vi "PID Drive.vi"(6 "Rotation":dbl, 7 "Gyro Angle":dbl, 8 "error in (no error)":errorcluster, 9 "Y":dbl, 10 "X":dbl, 11 "RobotDriveDevRef 2":T2={"DevStatus"={"status"=FALSE, "code"=0, "source"=""}, "Motors[]"=[{"DeviceStatus"={"status"=FALSE, "code"=0, "source"=""}, "Type"=enum."PWM", "PWM"={"Digital Module"=enum."Digital Module 1", "PWM Channel"=enum."PWM 2", "DeadBand"={"Name"="Victor", "maxPositivePwm"=208, "minPositivePwm"=129, "centerPwm"=128, "maxNegativePwm"=127, "minNegativePwm"=54, "angularRange"=0}}, "CAN"={"Device Number"=0, "Control Mode"=enum."Percent VBus", "Semaphore"=refnum, "Max Vout"=0.0}, "Invert"=FALSE, "TransformRef"=refnum, "InvTransformRef"=refnum}, {"DeviceStatus"={"status"=FALSE, "code"=0, "source"=""}, "Type"=enum."PWM", "PWM"={"Digital Module"=enum."Digital Module 1", "PWM Channel"=enum."PWM 1", "DeadBand"={"Name"="Victor", "maxPositivePwm"=208, "minPositivePwm"=129, "centerPwm"=128, "maxNegativePwm"=127, "minNegativePwm"=54, "angularRange"=0}}, "CAN"={"Device Number"=0, "Control Mode"=enum."Percent VBus", "Semaphore"=refnum, "Max Vout"=0.0}, "Invert"=TRUE, "TransformRef"=refnum, "InvTransformRef"=refnum}, {"DeviceStatus"={"status"=FALSE, "code"=0, "source"=""}, "Type"=enum."PWM", "PWM"={"Digital Module"=enum."Digital Module 1", "PWM Channel"=enum."PWM 4", "DeadBand"={"Name"="Victor", "maxPositivePwm"=208, "minPositivePwm"=129, "centerPwm"=128, "maxNegativePwm"=127, "minNegativePwm"=54, "angularRange"=0}}, "CAN"={"Device Number"=0, "Control Mode"=enum."Percent VBus", "Semaphore"=refnum, "Max Vout"=0.0}, "Invert"=FALSE, "TransformRef"=refnum, "InvTransformRef"=refnum}, {"DeviceStatus"={"status"=FALSE, "code"=0, "source"=""}, "Type"=enum."PWM", "PWM"={"Digital Module"=enum."Digital Module 1", "PWM Channel"=enum."PWM 3", "DeadBand"={"Name"="Victor", "maxPositivePwm"=208, "minPositivePwm"=129, "centerPwm"=128, "maxNegativePwm"=127, "minNegativePwm"=54, "angularRange"=0}}, "CAN"={"Device Number"=0, "Control Mode"=enum."Percent VBus", "Semaphore"=refnum, "Max Vout"=0.0}, "Invert"=TRUE, "TransformRef"=refnum, "InvTransformRef"=refnum}], "Square Inputs"=TRUE, "Max Output"=1.0, "Isochronous"=FALSE}) -> (0 "error out":errorcluster, 2 "Motor Values":dbl[](array[numeric])=[0.0, -0.0, 0.0, -0.0], 3 "RobotDriveDevRef":T2={"DevStatus"={"status"=FALSE, "code"=0, "source"=""}, "Motors[]"=[{"DeviceStatus"={"status"=FALSE, "code"=0, "source"=""}, "Type"=enum."PWM", "PWM"={"Digital Module"=enum."Digital Module 1", "PWM Channel"=enum."PWM 2", "DeadBand"={"Name"="Victor", "maxPositivePwm"=208, "minPositivePwm"=129, "centerPwm"=128, "maxNegativePwm"=127, "minNegativePwm"=54, "angularRange"=0}}, "CAN"={"Device Number"=0, "Control Mode"=enum."Percent VBus", "Semaphore"=refnum, "Max Vout"=0.0}, "Invert"=FALSE, "TransformRef"=refnum, "InvTransformRef"=refnum}, {"DeviceStatus"={"status"=FALSE, "code"=0, "source"=""}, "Type"=enum."PWM", "PWM"={"Digital Module"=enum."Digital Module 1", "PWM Channel"=enum."PWM 1", "DeadBand"={"Name"="Victor", "maxPositivePwm"=208, "minPositivePwm"=129, "centerPwm"=128, "maxNegativePwm"=127, "minNegativePwm"=54, "angularRange"=0}}, "CAN"={"Device Number"=0, "Control Mode"=enum."Percent VBus", "Semaphore"=refnum, "Max Vout"=0.0}, "Invert"=TRUE, "TransformRef"=refnum, "InvTransformRef"=refnum}, {"DeviceStatus"={"status"=FALSE, "code"=0, "source"=""}, "Type"=enum."PWM", "PWM"={"Digital Module"=enum."Digital Module 1", "PWM Channel"=enum."PWM 4", "DeadBand"={"Name"="Victor", "maxPositivePwm"=208, "minPositivePwm"=129, "centerPwm"=128, "maxNegativePwm"=127, "minNegativePwm"=54, "angularRange"=0}}, "CAN"={"Device Number"=0, "Control Mode"=enum."Percent VBus", "Semaphore"=refnum, "Max Vout"=0.0}, "Invert"=FALSE, "TransformRef"=refnum, "InvTransformRef"=refnum}, {"DeviceStatus"={"status"=FALSE, "code"=0, "source"=""}, "Type"=enum."PWM", "PWM"={"Digital Module"=enum."Digital Module 1", "PWM Channel"=enum."PWM 3", "DeadBand"={"Name"="Victor", "maxPositivePwm"=208, "minPositivePwm"=129, "centerPwm"=128, "maxNegativePwm"=127, "minNegativePwm"=54, "angularRange"=0}}, "CAN"={"Device Number"=0, "Control Mode"=enum."Percent VBus", "Semaphore"=refnum, "Max Vout"=0.0}, "Invert"=TRUE, "TransformRef"=refnum, "InvTransformRef"=refnum}], "Square Inputs"=TRUE, "Max Output"=1.0, "Isochronous"=FALSE})   [LabVIEW 2013]
uses:
  <vilib>/Rock Robotics/WPI/RobotDrive/WPI_RobotDriveDevRef.ctl
  <vilib>/Rock Robotics/WPI/MotorControl/WPI_MotorControlDeviceRef.ctl
  <vilib>/Rock Robotics/SystemInterfaces/Typedef/FPGA_TypedefDigitalModule.ctl
  <vilib>/Rock Robotics/SystemInterfaces/DIO/FPGA_DIOPWMChannel.ctl
  <vilib>/Rock Robotics/WPI/PWM/WPI_PWMDeadband.ctl
  <vilib>/Rock Robotics/WPI/CAN/Jaguar/SubVIs/WPI_CANJaguar_ControlMode.ctl
  <vilib>/Rock Robotics/WPI/PWM/WPI_PWMTransform_ConPane.ctl
  <vilib>/Rock Robotics/SystemInterfaces/NetworkCommunication/NetComm_UsageReport_ResourceType.ctl
  <vilib>/Rock Robotics/WPI/RobotDrive/WPI_RobotDriveMotorSelectorEnum.ctl
  <vilib>/addons/control/pid/pid.llb/PID (DBL).vi
  <vilib>/Rock Robotics/WPI/RobotDrive/WPI_RobotDriveSafetyCheck.vi
  <vilib>/addons/control/pid/NI_PID_pid.lvlib
panel:
  in  "Encoder Max":dbl=200.0
  in  "Back Right":T1={"proportional gain (Kc)"=0.01, "integral time (Ti, min)"=0.0, "derivative time (Td, min)"=0.0} {"derivative time (Td, min)" format="%.3f"; "integral time (Ti, min)" format="%.3f"; "proportional gain (Kc)" format="%.3f"}
  in  "Front Right":T1={"proportional gain (Kc)"=1.0, "integral time (Ti, min)"=0.0, "derivative time (Td, min)"=0.0} {"derivative time (Td, min)" format="%.3f"; "integral time (Ti, min)" format="%.3f"; "proportional gain (Kc)" format="%.3f"}
  in  "Back Left":T1={"proportional gain (Kc)"=0.01, "integral time (Ti, min)"=0.0, "derivative time (Td, min)"=0.0} {"derivative time (Td, min)" format="%.3f"; "integral time (Ti, min)" format="%.3f"; "proportional gain (Kc)" format="%.3f"}
  in  "Front Left":T1={"proportional gain (Kc)"=0.01, "integral time (Ti, min)"=0.0, "derivative time (Td, min)"=0.0} {"derivative time (Td, min)" format="%.3f"; "integral time (Ti, min)" format="%.3f"; "proportional gain (Kc)" format="%.3f"}
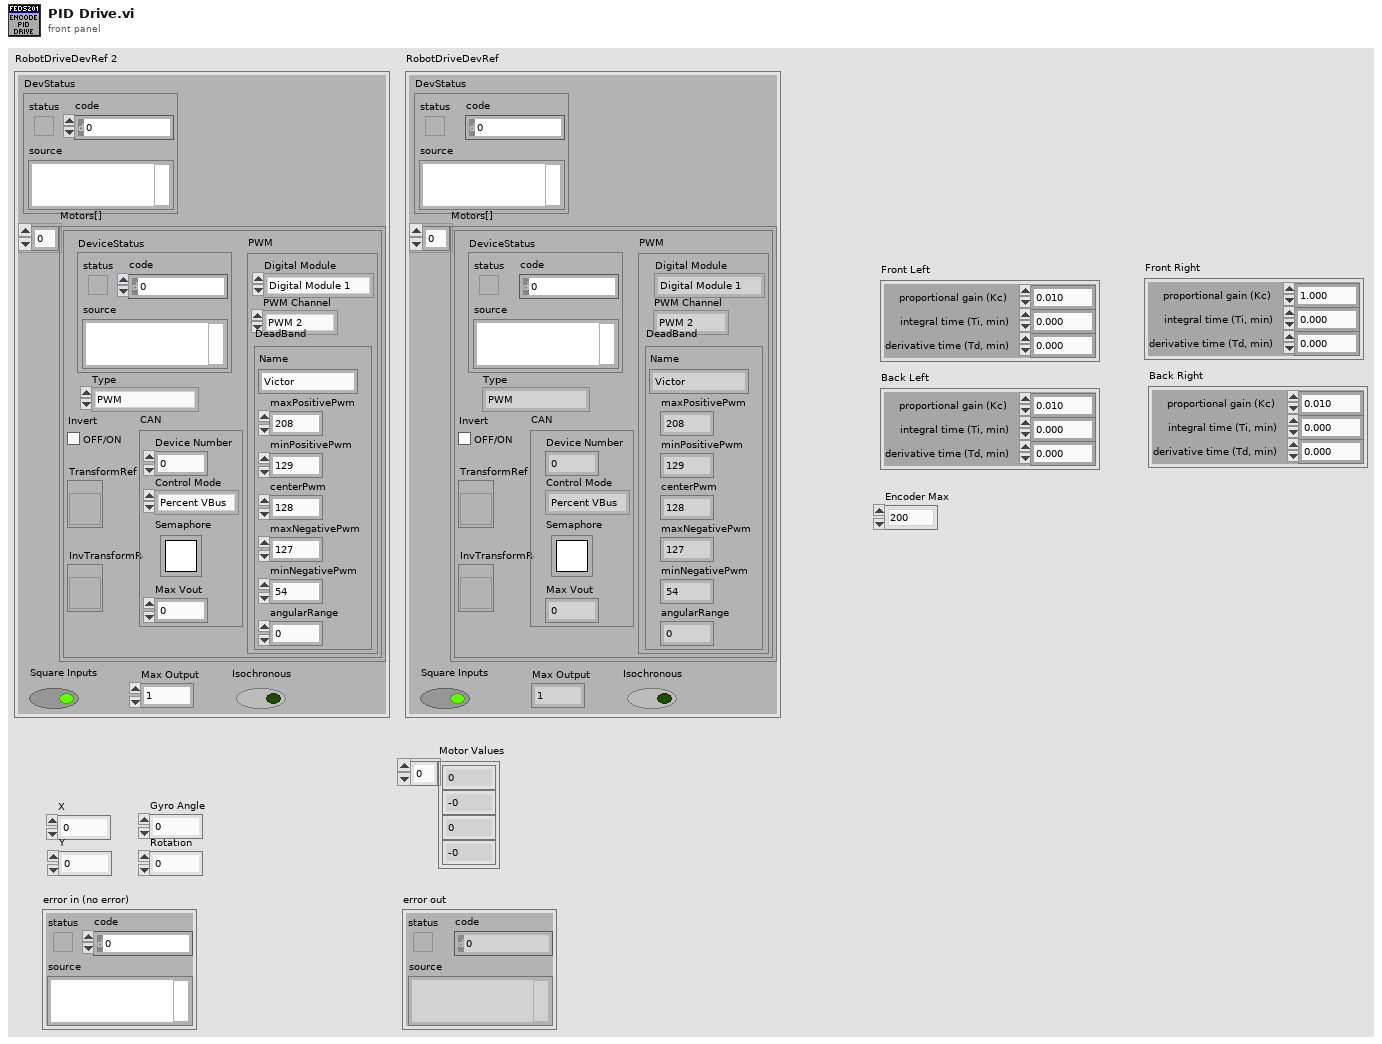
[diagram p1: front panel]
types:
  T1 = cluster{"proportional gain (Kc)":dbl, "integral time (Ti, min)":dbl, "derivative time (Td, min)":dbl}
  T2 = typedef "WPI_RobotDriveDevRef.ctl" = cluster{"DevStatus":errorcluster, "Motors[]":T3[], "Square Inputs":bool, "Max Output":dbl, "Isochronous":bool}
  T3 = typedef "WPI_MotorControlDeviceRef.ctl" = cluster{"DeviceStatus":errorcluster, "Type":enum16{"PWM", "CAN"}, "PWM":cluster{"Digital Module":T4, "PWM Channel":T5, "DeadBand":T6}, "CAN":cluster{"Device Number":u8, "Control Mode":T7, "Semaphore":T8, "Max Vout":dbl}, "Invert":bool, "TransformRef":T9, "InvTransformRef":T9}
  T4 = typedef "FPGA_TypedefDigitalModule.ctl" = enum16{"Digital Module 1", "Digital Module 2"}
  T5 = typedef "FPGA_DIOPWMChannel.ctl" = enum8{"PWM 1", "PWM 2", "PWM 3", "PWM 4", "PWM 5", "PWM 6", "PWM 7", "PWM 8", "PWM 9", "PWM 10", "Invalid"}
  T6 = typedef "WPI_PWMDeadband.ctl" = cluster{"Name":string, "maxPositivePwm":i32, "minPositivePwm":i32, "centerPwm":i32, "maxNegativePwm":i32, "minNegativePwm":i32, "angularRange":u16}
  T7 = typedef "WPI_CANJaguar_ControlMode.ctl" = enum8{"Percent VBus", "Current", "Speed", "Position", "Voltage"}
  T8 = typedef "Semaphore RefNum" = refnum<k1>
  T9 = typedef "WPI_PWMTransform_ConPane.ctl" = refnum<vi>
  T10 = typedef "NetComm_UsageReport_ResourceType.ctl" = enum8{"Controller", "Module", "Language", "CANPlugin", "Accelerometer", "ADXL345", "AnalogChannel", "AnalogTrigger", "AnalogTriggerOutput", "CANJaguar", "Compressor", "Counter", "Dashboard", "DigitalInput", "DigitalOutput", "DriverStationCIO", "DriverStationEIO", "DriverStationLCD", "Encoder", "GearTooth", "Gyro", "I2C", "Framework", "Jaguar", "Joystick", "Kinect", "KinectStick", "PIDController", "Preferences", "PWM", "Relay", "RobotDrive", "SerialPort", "Servo", "Solenoid", "SPI", "Task", "Ultrasonic", "Victor", "Button", "Command", "AxisCamera", "PCVideoServer", "SmartDashboard", "Talon", "HiTechnicColorSensor", "HiTechnicAccel", "HiTechnicCompass", "SRF08"}
  T11 = typedef "WPI_RobotDriveMotorSelectorEnum.ctl" = enum16{"Rear Left Motor", "Rear Right Motor", "Front Left Motor", "Front Right Motor"}
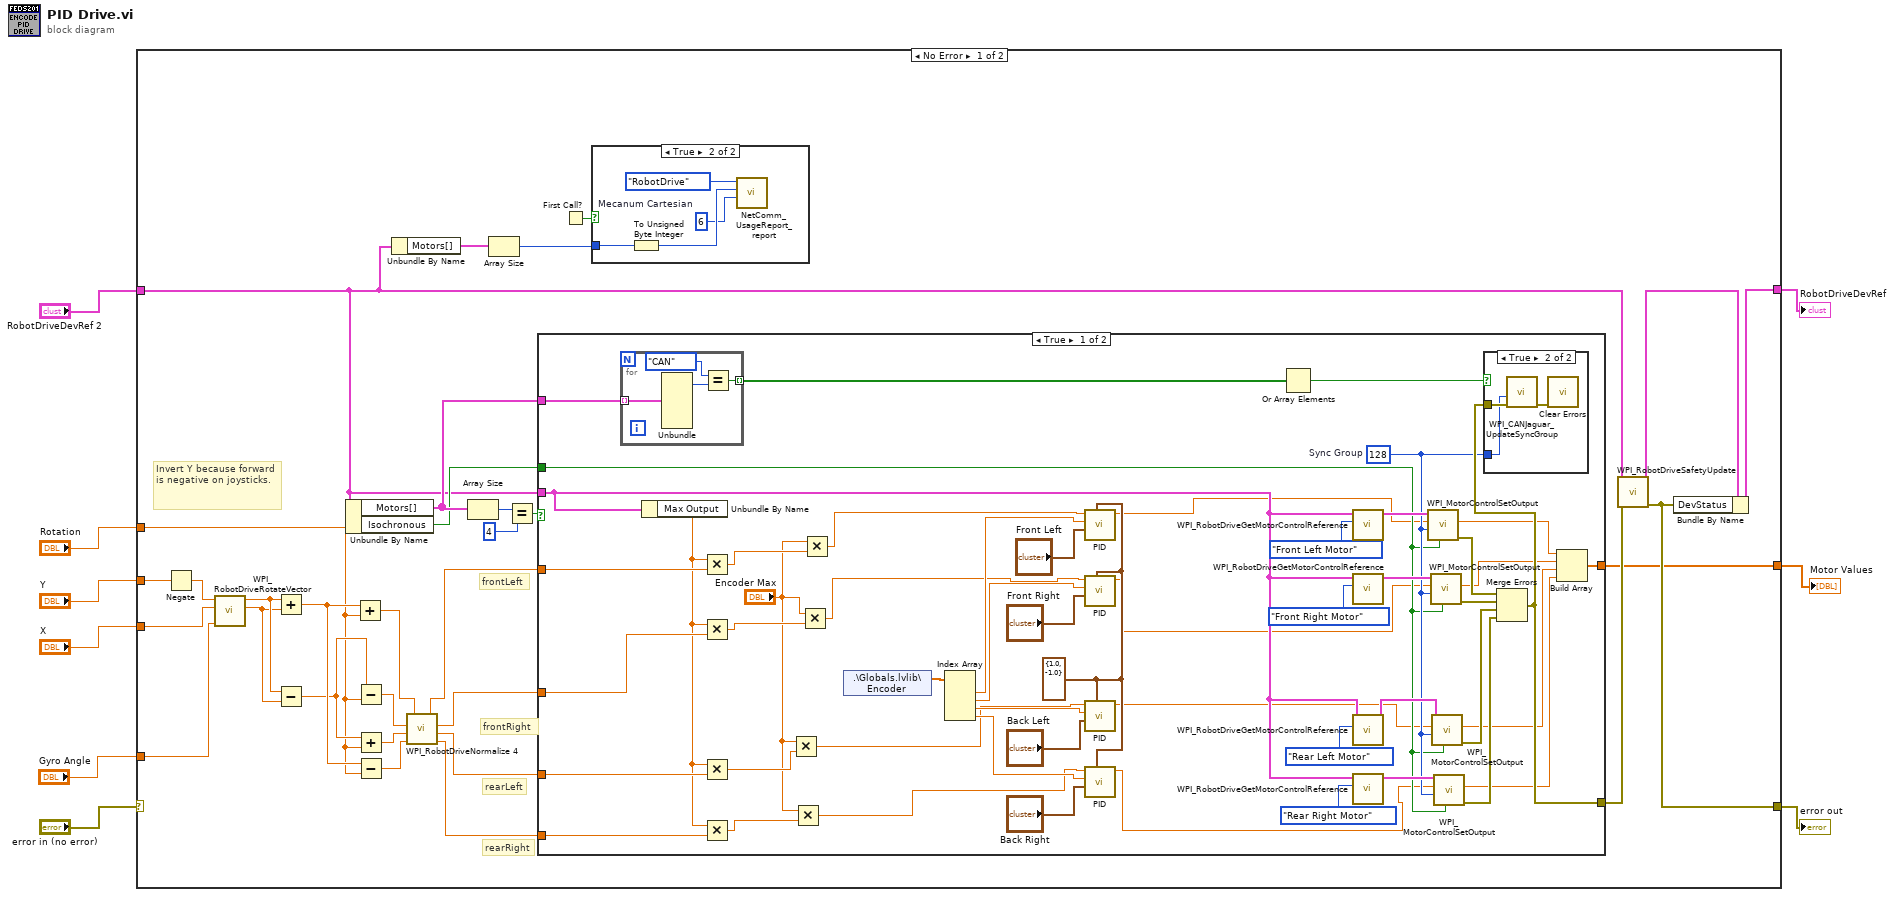
[diagram p0: block diagram]
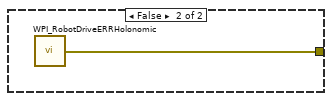
[diagram p4: hidden frame]
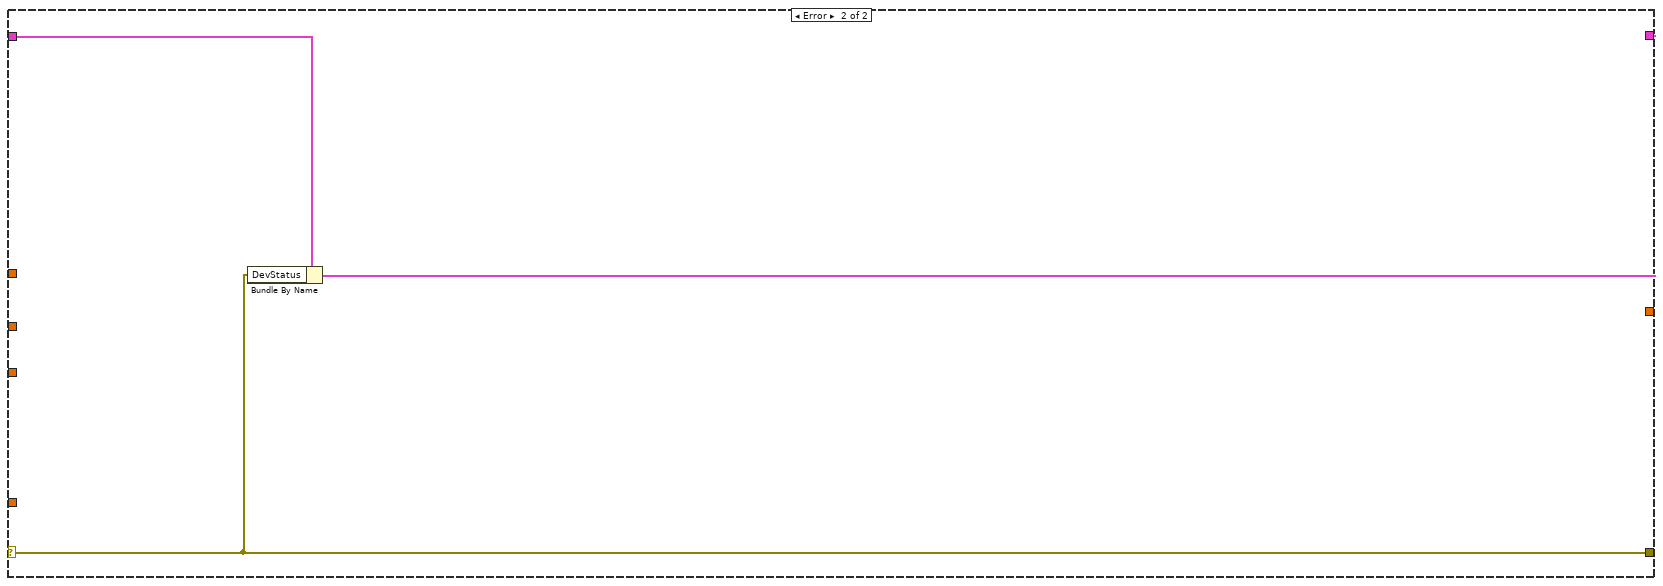
[diagram p5: hidden frame]
diagram:
  n1 = case shown="No Error" "error in (no error)" {
    selector: "error in (no error)" -> [_ w105]
    tunnel: "Y" -> [w22 _]
    tunnel: "X" -> [w27 _]
    tunnel: "RobotDriveDevRef 2" -> [w11 w107]
    tunnel: [w37 w106] -> w5
    tunnel: [w17 w105] -> w4
    tunnel: "Rotation" -> [w28 _]
    tunnel: "Gyro Angle" -> [w21 _]
    tunnel: [w10 _] -> w1
    frame No Error {
      # "Invert Y because forward is negative on joysticks."
      # "rearLeft"
      # "frontRight"
      # "rearRight"
      # "frontLeft"
      n2 = Negate(x=w22) -> (-x=w20:dbl)
      n3 = call <vilib>:"WPI_RobotDriveRotateVector.vi"("Angle"=w21, "X"=w27, "Y"=w20) -> ("X'"=w35:dbl, "Y'"=w36:dbl)  [unwired: 7 out]
      n4 = Add(x=w36, y=w35) -> (x+y=w33:dbl)
      n5 = Subtract(x=w36, y=w35) -> (x-y=w31:dbl)
      n6 = Unbundle By Name(w11) -> ("Motors[]"=w16:T3[], "Isochronous"=w15:bool)
      n7 = Add(x=w33, y=w28) -> (x+y=w29:dbl)
      n8 = Subtract(x=w31, y=w28) -> (x-y=w30:dbl)
      n9 = Add(x=w31, y=w28) -> (x+y=w32:dbl)
      n10 = Subtract(x=w33, y=w28) -> (x-y=w34:dbl)
      n11 = Unbundle By Name(w11) -> ("Motors[]"=w13:T3[])
      n12 = call <vilib>:"WPI_RobotDriveNormalize 4.vi"("D"=w34, "C"=w32, "B"=w30, "A"=w29) -> ("D'"=w24:dbl, "C'"=w23:dbl, "B'"=w25:dbl, "A'"=w26:dbl)
      n13 = Array Size(array=w16) -> (size(s)=w40:i32)
      n14 = Array Size(array=w13) -> (size(s)=w12:i32)
      n15 = Equal?(x=w40, y=4) -> (x = y?=w38:bool)
      n16 = case shown="True" w38 {
        tunnel: w26 -> [w96 _]
        tunnel: w25 -> [w95 _]
        tunnel: w11 -> [w84 _]
        tunnel: [w75 w104] -> w19
        tunnel: w23 -> [w90 _]
        tunnel: w24 -> [w89 _]
        tunnel: w16 -> [w76 _]
        tunnel: w15 -> [w73 _]
        tunnel: [w71 _] -> w10
        frame True {
          w62 = cluster{"output high":dbl, "output low":dbl} {"output high"=1.0, "output low"=-1.0} ("output range")
          w74 = u8 128  # Sync Group
          n17 = for {
            tunnel: w76 -> [w100] mode=indexing
            tunnel: [w97] -> w77 mode=indexing
            n18 = Unbundle(w100) -> ("Type"=w99:enum16{"PWM", "CAN"})  [unwired: 6 out]
            n19 = Equal?(x=enum16{"PWM", "CAN"}."CAN" ("Type"), y=w99) -> (x = y?=w97:bool)
          }
          n20 = Unbundle By Name(w84) -> ("Max Output"=w83:dbl)
          n21 = Multiply(x=w83, y=w96) -> (x*y=w53:dbl)
          n22 = Multiply(x=w83, y=w95) -> (x*y=w52:dbl)
          n23 = Multiply(x=w83, y=w90) -> (x*y=w51:dbl)
          n24 = Multiply(x=w83, y=w89) -> (x*y=w50:dbl)
          n25 = Multiply(x="Encoder Max", y=w51) -> (x*y=w48:dbl)
          n26 = Multiply(x="Encoder Max", y=w50) -> (x*y=w49:dbl)
          n27 = Multiply(x="Encoder Max", y=w52) -> (x*y=w47:dbl)
          n28 = Multiply(x="Encoder Max", y=w53) -> (x*y=w46:dbl)
          n29 = shared-variable ".\\Globals.lvlib\\Encoder"() -> (w67:dbl[])  [unwired: 1 in, 1 out]
          n30 = Index Array(array=w67) -> (element #1=w66:dbl, element #2=w65:dbl, element #3=w64:dbl, element #4=w63:dbl)  [unwired: 4 in]
          n31 = call-poly <vilib>:"PID.vi"("output range"=w62, "PID gains"="Front Left", "process variable"=w66, "setpoint"=w46) -> ("output"=w57:dbl)  [unwired: 6 in, 1 out]
          n32 = call-poly <vilib>:"PID.vi"("output range"=w62, "PID gains"="Front Right", "process variable"=w65, "setpoint"=w47) -> ("output"=w56:dbl)  [unwired: 6 in, 1 out]
          n33 = call-poly <vilib>:"PID.vi"("output range"=w62, "PID gains"="Back Left", "process variable"=w64, "setpoint"=w48) -> ("output"=w55:dbl)  [unwired: 6 in, 1 out]
          n34 = call-poly <vilib>:"PID.vi"("output range"=w62, "PID gains"="Back Right", "process variable"=w63, "setpoint"=w49) -> ("output"=w54:dbl)  [unwired: 6 in, 1 out]
          n35 = Or Array Elements(Boolean array=w77) -> (logical OR=w78:bool)
          n36 = call <vilib>:"WPI_RobotDriveGetMotorControlReference.vi"("MotorIndex"=WPI_RobotDriveMotorSelectorEnum."Front Left Motor", "RobotDriveDevRef"=w84) -> ("MotorControlDeviceRef"=w94:T3)  [unwired: 9 out]
          n37 = call <vilib>:"WPI_RobotDriveGetMotorControlReference.vi"("MotorIndex"=WPI_RobotDriveMotorSelectorEnum."Front Right Motor", "RobotDriveDevRef"=w84) -> ("MotorControlDeviceRef"=w92:T3)  [unwired: 9 out]
          n38 = call <vilib>:"WPI_RobotDriveGetMotorControlReference.vi"("MotorIndex"=WPI_RobotDriveMotorSelectorEnum."Rear Left Motor", "RobotDriveDevRef"=w84) -> ("MotorControlDeviceRef"=w93:T3)  [unwired: 9 out]
          n39 = call <vilib>:"WPI_RobotDriveGetMotorControlReference.vi"("MotorIndex"=WPI_RobotDriveMotorSelectorEnum."Rear Right Motor", "RobotDriveDevRef"=w84) -> ("MotorControlDeviceRef"=w91:T3)  [unwired: 9 out]
          n40 = call <vilib>:"WPI_MotorControlSetOutput.vi"("Isochronous"=w73, "Sync Group"=w74, "Output"=w57, "MotorControlDevRef"=w94) -> ("error out"=w79:errorcluster, "Motor Output"=w72:dbl)  [unwired: 1 in, 5 out]
          n41 = call <vilib>:"WPI_MotorControlSetOutput.vi"("Isochronous"=w73, "Sync Group"=w74, "Output"=w56, "MotorControlDevRef"=w92) -> ("error out"=w80:errorcluster, "Motor Output"=w70:dbl)  [unwired: 1 in, 5 out]
          n42 = call <vilib>:"WPI_MotorControlSetOutput.vi"("Isochronous"=w73, "Sync Group"=w74, "Output"=w55, "MotorControlDevRef"=w93) -> ("error out"=w81:errorcluster, "Motor Output"=w69:dbl)  [unwired: 1 in, 5 out]
          n43 = call <vilib>:"WPI_MotorControlSetOutput.vi"("Isochronous"=w73, "Sync Group"=w74, "Output"=w54, "MotorControlDevRef"=w91) -> ("error out"=w82:errorcluster, "Motor Output"=w68:dbl)  [unwired: 1 in, 5 out]
          n44 = Merge Errors(w79, w80, w81, w82) -> (w75:errorcluster)
          n45 = case shown="True" w78 {
            tunnel: w75 -> [_ w102]
            tunnel: w74 -> [_ w101]
            frame False {
            }
            frame True {
              n46 = call <vilib>:"WPI_CANJaguar_UpdateSyncGroup.vi"("error in (no error)"=w102, "Sync Group"=w101) -> ("error out"=w103:errorcluster)  [unwired: 9 out]
              n47 = call <vilib>:"Clear Errors.vi"("error in (no error)"=w103) -> ()  [unwired: 7 out]
            }
          }
          n48 = Build Array(w72, w70, w69, w68) -> (w71:dbl[])
        }
        frame False {
          n49 = call <vilib>:"WPI_RobotDriveERRHolonomic.vi"() -> ("error out"=w104:errorcluster)
        }
      }
      n50 = First Call?() -> (First Call?: T/F=w14:bool)
      n51 = case shown="True" w14 {
        tunnel: w12 -> [_ w43]
        frame False {
        }
        frame True {
          w41 = u8 6  # Mecanum Cartesian
          n52 = To Unsigned Byte Integer(number=w43) -> (unsigned 8bit integer=w42:u8)
          n53 = call <vilib>:"NetComm_UsageReport_report.vi"("Context"=w41, "Instance Number"=w42, "Resource Type"=NetComm_UsageReport_ResourceType."RobotDrive") -> ()  [unwired: 9 in]
        }
      }
      n54 = call <vilib>:"WPI_RobotDriveSafetyUpdate.vi"("error in (no error)"=w19, "RobotDriveDevRef"=w11) -> ("error out"=w17:errorcluster, "RobotDriveDevRef"=w18:T2)  [unwired: 8 out]
      n55 = Bundle By Name(cluster=w18, "DevStatus"=w17) -> (w37:T2)
    }
    frame Error {
      n56 = Bundle By Name(cluster=w107, "DevStatus"=w105) -> (w106:T2)
    }
  }
  "error out" <- w4
  "RobotDriveDevRef" <- w5
  "Motor Values" <- w1
